vi "PID Output Rate Limiter Inn.vi"(7 "reinitialize? (F)":bool, 8 "dt (s)":dbl=0.1 format="%.2f", 9 "output rate (EGU/s)":dbl=1.0 format="%.2f", 10 "output old":dbl format="%.2f", 11 "input (controller output)":dbl format="%.2f") -> (3 "output":dbl format="%.2f")   [LabVIEW 2019, in "control.lvlib"]
uses:
  control.lvlib
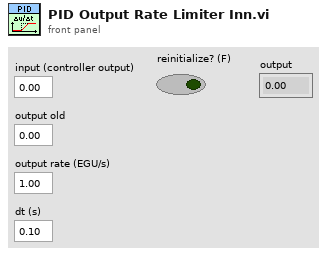
[diagram p1: front panel]
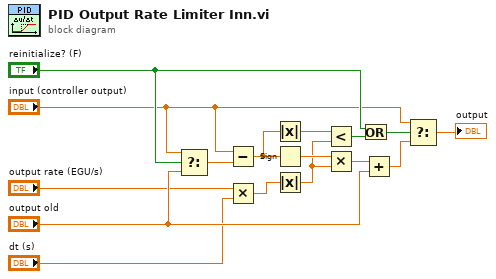
[diagram p0: block diagram]
diagram:
  n1 = Select(t="input (controller output)", s="reinitialize? (F)", f="output old") -> (s? t:f=w9:dbl)
  n2 = Subtract(x="input (controller output)", y=w9) -> (x-y=w12:dbl)
  n3 = Multiply(x="output rate (EGU/s)", y="dt (s)") -> (x*y=w14:dbl)
  n4 = Absolute Value(x=w12) -> (abs(x)=w7:dbl)
  n5 = Sign(1:w12) -> (0:w10:dbl)
  n6 = Absolute Value(x=w14) -> (abs(x)=w6:dbl)
  n7 = Less?(x=w7, y=w6) -> (x < y?=w13:bool)
  n8 = Multiply(x=w10, y=w6) -> (x*y=w8:dbl)
  n9 = Or(x="reinitialize? (F)", y=w13) -> (x .or. y?=w5:bool)
  n10 = Add(x=w8, y="output old") -> (x+y=w11:dbl)
  n11 = Select(t="input (controller output)", s=w5, f=w11) -> (s? t:f=→"output":dbl)
